vi "Write Data to VS Engine.vi"(7 "Write to VS Engine FIFO":refnum<k33>, 8 "error in":errorcluster, 10 "Values":dbl[](array[numeric]), 11 "Result Ch Data Refs":T1[](array[typedef]) format="%.0x") -> (0 "error out":errorcluster, 1 "Read Occured":bool, 2 "Values out":dbl[](array[numeric]), 3 "Result Ch Data Refs out":T1[](array[typedef]) format="%.0x")   [LabVIEW 2015, in "Waveform-Processing-Custom-Device Engine.lvlib" / "Inline Async API.lvlib"]
uses:
  Inline Async API.lvlib
  Built/Waveform-Processing-Custom-Device/Waveform-Processing-Custom-Device Engine Windows.llb/Data Reference.ctl
  Built/Waveform-Processing-Custom-Device/c/Waveform-Processing-Custom-Device Engine Pharlap.llb/Global Data Refs.vi
  <vilib>/NI VeriStand/Custom Device API/Custom Device API.lvlib
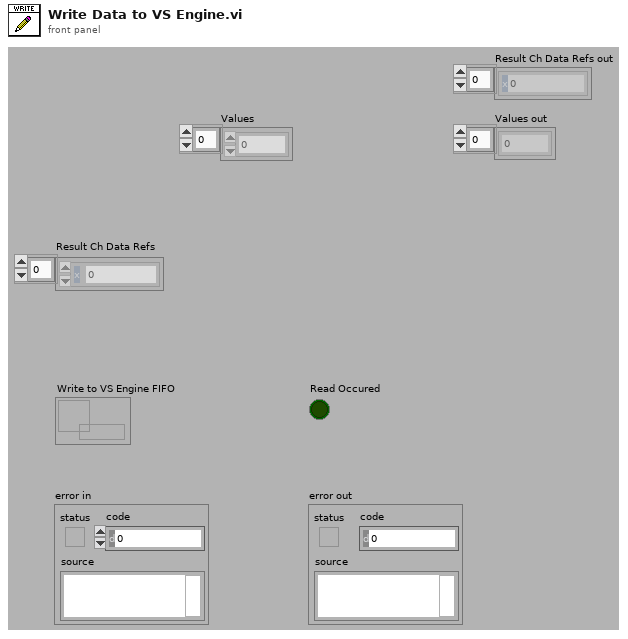
[diagram p1: front panel]
types:
  T1 = typedef "Custom Device API.lvlib/Data Reference.ctl" = i32
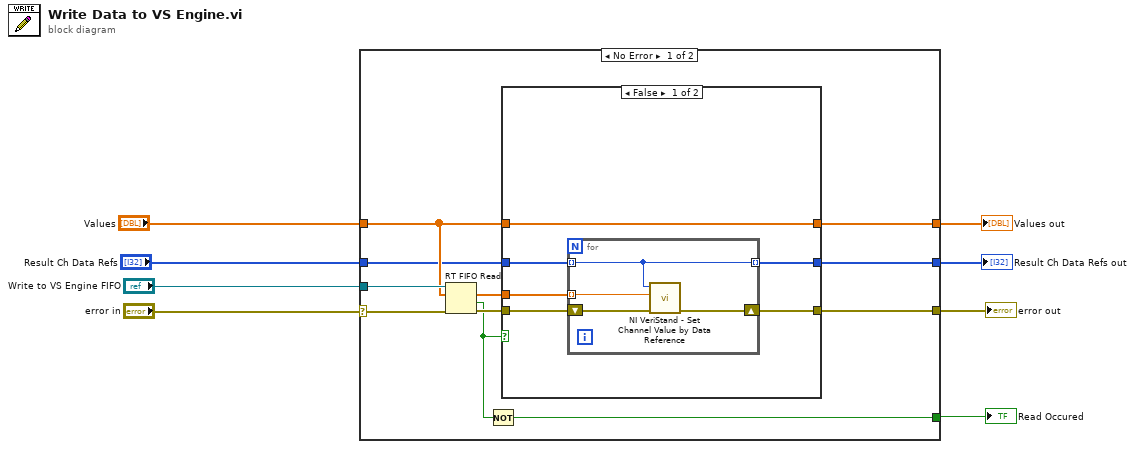
[diagram p0: block diagram]
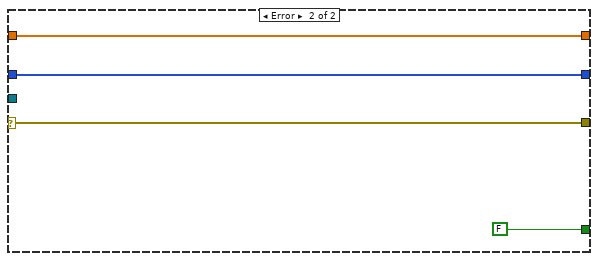
[diagram p3: hidden frame]
diagram:
  n1 = case shown="No Error" "error in" {
    selector: "error in" -> [w16 w36]
    tunnel: [w19 w36] -> w8
    tunnel: [w12 w34] -> w3
    tunnel: [w14 FALSE ("C Read Occured?")] -> w7
    tunnel: "Write to VS Engine FIFO" -> [w13 _]
    tunnel: "Values" -> [w11 w34]
    tunnel: "Result Ch Data Refs" -> [w10 w33]
    tunnel: [w9 w33] -> w1
    frame No Error {
      n2 = RT FIFO Read(0:w13, 1:w11, 3:w16) -> (9:w17:dbl[], 10:w15:bool, 11:w18:errorcluster)  [unwired: 1 in, 2 out]
      n3 = Not(x=w15) -> (.not. x?=w14:bool)
      n4 = case shown="False" w15 {
        tunnel: w18 -> [w25 w32]
        tunnel: w17 -> [w21 _]
        tunnel: [w23 w32] -> w19
        tunnel: [w20 w30] -> w12
        tunnel: w11 -> [w20 w30]
        tunnel: w10 -> [w24 w31]
        tunnel: [w22 w31] -> w9
        frame False {
          n5 = for {
            tunnel: w24 -> [w26] mode=indexing
            tunnel: [w26] -> w22 mode=indexing
            shift-right: [w28] -> w23
            shift-left: w25 -> [w29]
            tunnel: w21 -> [w27] mode=indexing
            n6 = call <vilib>:"NI VeriStand - Set Channel Value by Data Reference.vi"("error in (no error)"=w29, "Value"=w27, "Data Reference in"=w26) -> ("error out"=w28:errorcluster)  [unwired: 8 in]
          }
        }
        frame True {
        }
      }
    }
    frame Error {
    }
  }
  "error out" <- w8
  "Read Occured" <- w7
  "Values out" <- w3
  "Result Ch Data Refs out" <- w1
